vi "Scaled Error Function Complement.vi"(3 "x":dbl) -> (1 "scaled erfc(x)":dbl)   [LabVIEW 2017, in "NI_AAL_MathFunc.lvlib"]
doc: "Computes the scaled complementary error function associated with a normal distribution."
uses:
  <vilib>/gmath/NI_AAL_MathFunc.lvlib
  <vilib>/gmath/NI_Gmath.lvlib
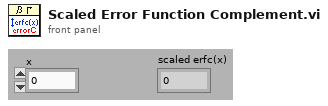
[diagram p1: front panel]
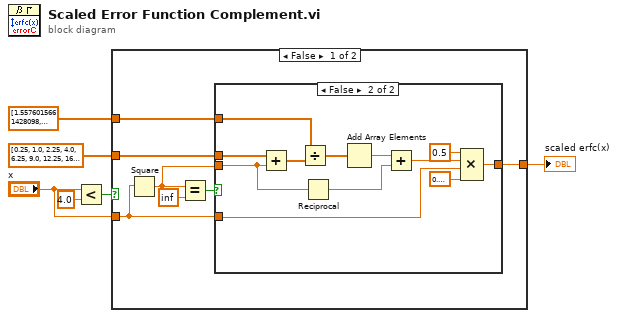
[diagram p0: block diagram]
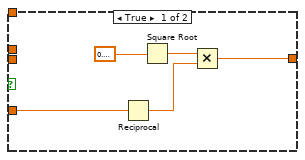
[diagram p2: hidden frame]
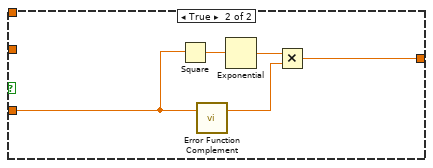
[diagram p3: hidden frame]
diagram:
  n1 = Less?(x="x", y=4.0) -> (x < y?=w1:bool)
  n2 = case shown="False" w1 {
    tunnel: [w11 w35] -> w4
    tunnel: dbl[] [0.25, 1.0, 2.25, 4.0, 6.25, 9.0, 12.25, 16.0, 20.25, 25.0] ("Array 2") -> [w13 _]
    tunnel: dbl[] [1.5576015661428098, 0.7357588823428847, 0.21079844912372867, 0.03663127777746836, 0.0038609082724554186, 0.0002468196081733591, 9.570234784258018e-06, 2.2507034943851823e-07, 3.2104561103712233e-09, 2.7775887729928042e-11] ("x*y") -> [w12 _]
    tunnel: "x" -> [w8 w31]
    frame False {
      n3 = Square(x=w8) -> (x^2=w7:dbl)
      n4 = Equal?(x=w7, y=inf) -> (x = y?=w9:bool)
      n5 = case shown="False" w9 {
        tunnel: w13 -> [_ w29]
        tunnel: w12 -> [_ w27]
        tunnel: w8 -> [w17 w21]
        tunnel: [w14 w20] -> w11
        tunnel: w7 -> [_ w19]
        frame True {
          n6 = Reciprocal(x=w17) -> (1/x=w15:dbl)
          n7 = Square Root(x=0.3183098861837907) -> (sqrt(x)=w16:dbl)
          n8 = Multiply(x=w16, y=w15) -> (x*y=w14:dbl)
        }
        frame False {
          n9 = Add(x=w29, y=w19) -> (x+y=w28:dbl[])
          n10 = Divide(x=w27, y=w28) -> (x/y=w30:dbl[])
          n11 = Reciprocal(x=w19) -> (1/x=w25:dbl)
          n12 = Add Array Elements(numeric array=w30) -> (sum=w22:dbl)
          n13 = Add(x=w22, y=w25) -> (x+y=w26:dbl)
          n14 = Compound Arithmetic op=MULTIPLY(0.5 ("value"), w26, w21, 0.3183098861837907) -> (w20:dbl)
        }
      }
    }
    frame True {
      n15 = Square(x=w31) -> (x^2=w34:dbl)
      n16 = call <vilib>:"Error Function Complement.vi"("x"=w31) -> ("1 - erf(x)"=w33:dbl)  [unwired: 2 out]
      n17 = Exponential(1:w34) -> (0:w32:dbl)
      n18 = Multiply(x=w32, y=w33) -> (x*y=w35:dbl)
    }
  }
  "scaled erfc(x)" <- w4
